vi "Broadcast Response.vi"(8 "error in (no error)":errorcluster, 9 "Acquired Result.lvclass":refnum<class "Acquired Result.lvclass">, 10 "Topic":string, 11 "Process Object in":refnum<class "Process Object.lvclass">) -> (0 "error out":errorcluster, 3 "Process Object out":refnum<class "Process Object.lvclass">)   [LabVIEW 2019, in "Process Object.lvclass"]
uses:
  Process Object.lvclass
  NHMFL_Core/Libraries/Instruments/Results/Acquired Result/Acquired Result.lvclass
  Process Object.lvclass/Process Object.ctl
  Read Broadcaster name.vi
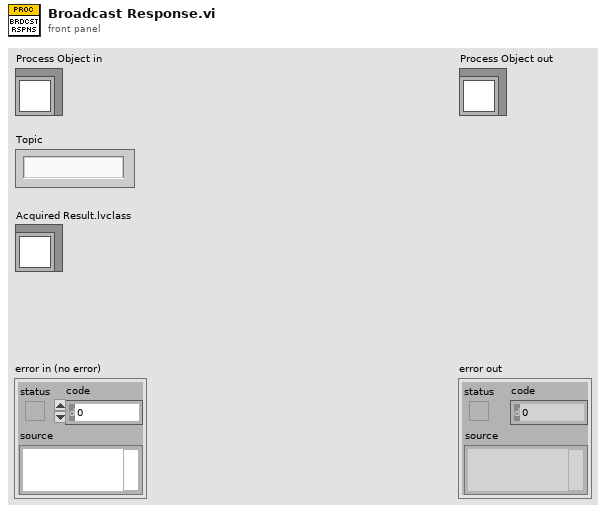
[diagram p1: front panel]
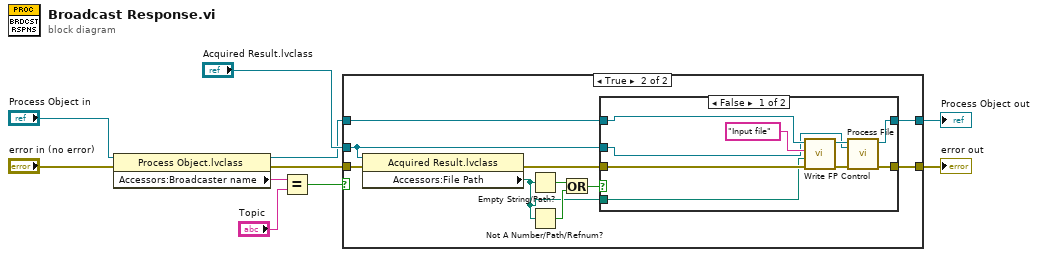
[diagram p0: block diagram]
diagram:
  n1 = property class="Process Object.lvclass"(reference="Process Object in", error in="error in (no error)") -> (reference out=w5:refnum<class "Process Object.lvclass">, error out=w4:errorcluster, "Accessors:Broadcaster name"=w9:string)
  n2 = Equal?(x=w9, y="Topic") -> (x = y?=w1:bool)
  n3 = case shown="True" w1 {
    tunnel: "Acquired Result.lvclass" -> [_ w14]
    tunnel: w4 -> [w12 w22]
    tunnel: w5 -> [w11 w21]
    tunnel: [w11 w19] -> w3
    tunnel: [w12 w18] -> w2
    frame False {
    }
    frame True {
      n4 = property class="Acquired Result.lvclass"(reference=w14, error in=w22) -> (error out=w20:errorcluster, "Accessors:File Path"=w13:path)  [unwired: 1 out]
      n5 = Empty String/Path?(string/path=w13) -> (empty?=w17:bool)
      n6 = Not A Number/Path/Refnum?(number/path/refnum=w13) -> (NaN/Path/Refnum?=w16:bool)
      n7 = Or(x=w17, y=w16) -> (x .or. y?=w15:bool)
      n8 = case shown="False" w15 {
        tunnel: w21 -> [w27 w33]
        tunnel: w20 -> [w31 w32]
        tunnel: [w25 w33] -> w19
        tunnel: [w24 w32] -> w18
        tunnel: w14 -> [w26 _]
        tunnel: w13 -> [w23 _]
        frame False {
          n9 = call-dynamic "Write FP Control.vi"("error in (no error)"=w31, "Control Value"=w23, "Control Name"="Input file", "Measure Object in"=w27) -> ("error out"=w29:errorcluster, "Measure Object out"=w28:refnum<class "Process Object.lvclass">)  [unwired: 6 in]
          n10 = call-dynamic "Process File.vi"("error in (no error)"=w29, "Result in"=w26, "Process Object in"=w28) -> ("error out"=w24:errorcluster, "Process Object out"=w25:refnum<class "Process Object.lvclass">)  [unwired: 6 in, 1 out]
        }
        frame True {
        }
      }
    }
  }
  "error out" <- w2
  "Process Object out" <- w3
